vi "ListDQMH_HighLevel_VIs.vi"(2 "Filter":string[](array[string])=["Validate DQMH Module", "Rename DQMH Module"], 11 "error in":errorcluster) -> (4 "Events_Name":string[](array[string]), 6 "Events_Tag":string[](array[string]), 8 "Module_Name":string[](array[string]), 10 "Module_Tag":string[](array[string]), 15 "error IO":errorcluster)   [LabVIEW 2012]
panel:
  # "Connector Pane"
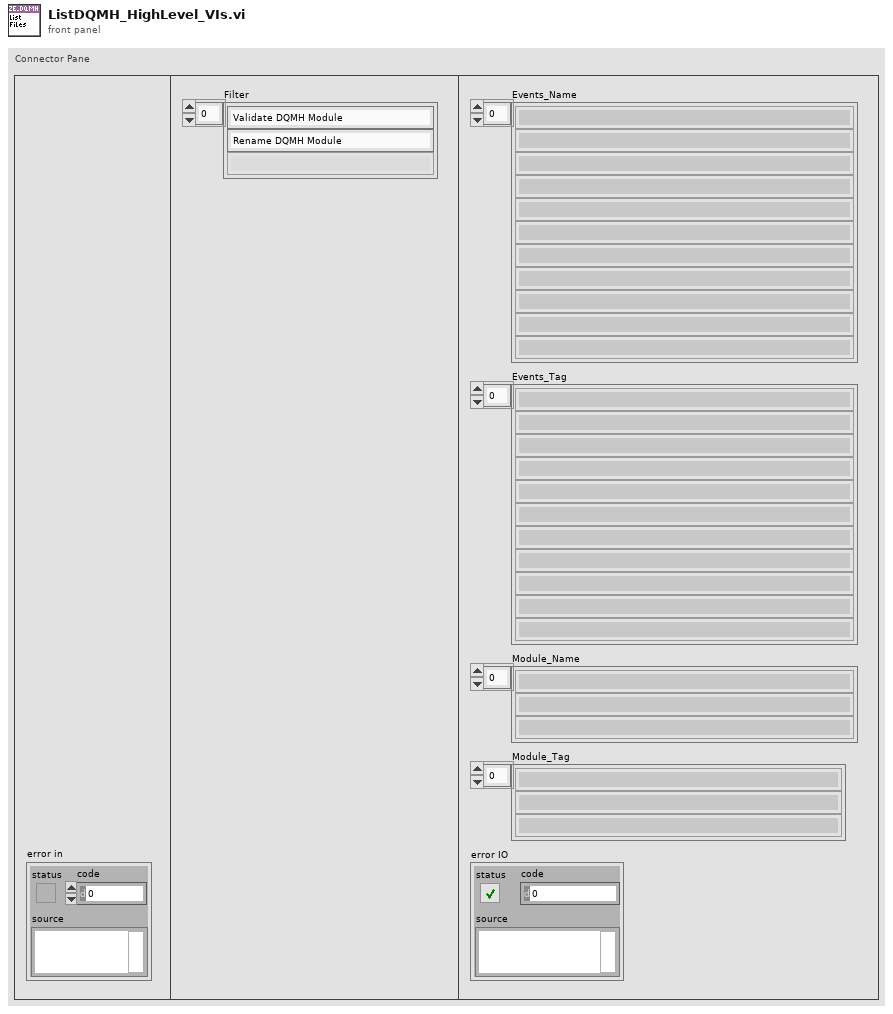
[diagram p1: front panel]
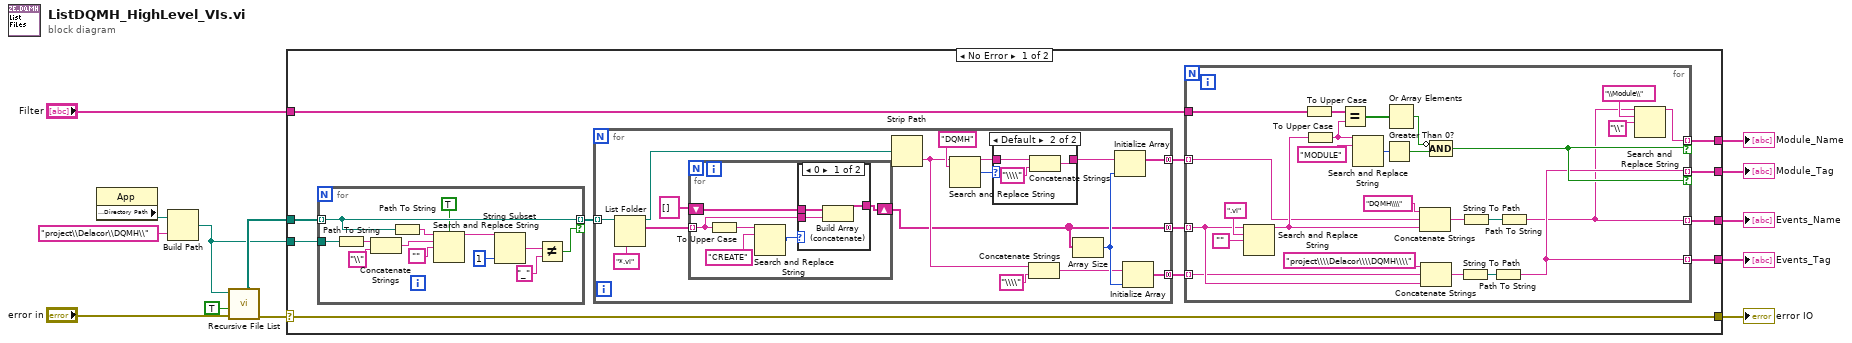
[diagram p0: block diagram]
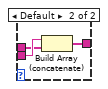
[diagram p2: hidden frame]
diagram:
  n1 = property class="App"() -> ("Application:Directory Path"=w11:path)  [unwired: 2 in, 2 out]
  n2 = Build Path(base path=w11, name or relative path="project\\Delacor\\DQMH\\") -> (appended path=w9:path)
  n3 = call <vilib>:"Recursive File List.vi"("error in (no error)"="error in", "Continue Recursing on Error? (F)"=TRUE, "Folder Path"=w9) -> ("error out"=w4:errorcluster, "All Folders"=w10:path[])  [unwired: 4 in, 3 out]
  n4 = case shown="No Error" w4 {
    selector: w4 -> [w18 w97]
    tunnel: w10 -> [w25 _]
    tunnel: w9 -> [w24 _]
    tunnel: [w21 _] -> w8
    tunnel: "Filter" -> [w20 _]
    tunnel: [w19 _] -> w1
    tunnel: [w18 w97] -> w5
    tunnel: [w17 _] -> w3
    tunnel: [w16 _] -> w2
    frame No Error {
      n5 = for {
        tunnel: w25 -> [w92] mode=indexing
        tunnel: [w92] -> w23 mode=indexing if=w93
        tunnel: w24 -> [w90]
        n6 = Path To String(path=w90) -> (string=w86:string)
        n7 = Concatenate Strings(w86, "\\" ("string")) -> (w85:string)
        n8 = Path To String(path=w92) -> (string=w91:string)
        n9 = Search and Replace String(case sensitive?=TRUE ("ignore case? (F)"), input string=w91, search string=w85, replace string="") -> (result string=w87:string)  [unwired: 4 in, 3 out]
        n10 = String Subset(string=w87, length (rest)=1 ("length (rest)")) -> (substring=w95:string)  [unwired: 1 in]
        n11 = Not Equal?(x=w95, y="_") -> (x != y?=w93:bool)
      }
      n12 = for {
        tunnel: w23 -> [w67] mode=indexing
        tunnel: [w52] -> w22 mode=concatenating
        tunnel: [w61] -> w15 mode=concatenating
        tunnel: [w56] -> w14 mode=concatenating
        n13 = List Folder(path=w67, pattern="*.vi") -> (path out=w59:path, filenames=w54:string[])  [unwired: 2 in, 2 out]
        n14 = for {
          tunnel: w54 -> [w71] mode=indexing
          shift-right: [w69] -> w52
          shift-left: string[] [] ("filenames") -> [w70]
          n15 = To Upper Case(1:w71) -> (0:w68:string)
          n16 = Search and Replace String(input string=w68, search string="CREATE") -> (number of replacements=w72:i32)  [unwired: 6 in, 3 out]
          n17 = case shown="0" w72 {
            tunnel: w71 -> [w76 w79]
            tunnel: w70 -> [w75 w78]
            tunnel: [w74 w77] -> w69
            frame 0 {
              n18 = Build Array (concatenate)(w75, w76) -> (w74:string[])
            }
            frame Default {
              n19 = Build Array (concatenate)(w79, w78) -> (w77:string[])
            }
          }
        }
        n20 = Strip Path(path=w59) -> (name=w55:string)  [unwired: 1 out]
        n21 = Search and Replace String(input string=w55, search string="DQMH") -> (result string=w63:string, number of replacements=w64:i32)  [unwired: 6 in, 2 out]
        n22 = case shown="Default" w64 {
          tunnel: w63 -> [w80 w83]
          tunnel: [w80 w81] -> w62
          frame 1.. {
          }
          frame Default {
            n23 = Concatenate Strings(w83, "\\\\" ("string")) -> (w81:string)
          }
        }
        n24 = Concatenate Strings(w55, "\\\\" ("string")) -> (w57:string)
        n25 = Array Size(array=w52) -> (size(s)=w60:i32)
        n26 = Initialize Array(w62, w60) -> (w61:string[])
        n27 = Initialize Array(w57, w60) -> (w56:string[])
      }
      n28 = for {
        tunnel: w22 -> [w36] mode=indexing
        tunnel: [w27] -> w21 mode=indexing
        tunnel: w20 -> [w48]
        tunnel: [w26] -> w19 mode=indexing if=w39
        tunnel: [w30] -> w17 mode=indexing if=w39
        tunnel: [w30] -> w16 mode=indexing
        tunnel: w15 -> [w37] mode=indexing
        tunnel: w14 -> [w35] mode=indexing
        n29 = Search and Replace String(input string=w36, search string=".vi", replace string="") -> (result string=w40:string)  [unwired: 5 in, 3 out]
        n30 = To Upper Case(1:w48) -> (0:w49:string[])
        n31 = To Upper Case(1:w40) -> (0:w46:string)
        n32 = Equal?(x=w49, y=w46) -> (x = y?=w47:bool[])
        n33 = Search and Replace String(input string=w46, search string="MODULE") -> (number of replacements=w44:i32)  [unwired: 6 in, 3 out]
        n34 = Greater Than 0?(x=w44) -> (x > 0?=w43:bool)
        n35 = Or Array Elements(Boolean array=w47) -> (logical OR=w42:bool)
        n36 = Concatenate Strings("DQMH\\\\" ("string"), w37, w40) -> (w34:string)
        n37 = Concatenate Strings("project\\\\Delacor\\\\DQMH\\\\" ("string"), w35, w36) -> (w33:string)
        n38 = Compound Arithmetic op=AND(invert w42, w43) -> (w39:bool)
        n39 = String To Path(string=w33) -> (path=w31:path)
        n40 = String To Path(string=w34) -> (path=w32:path)
        n41 = Path To String(path=w31) -> (string=w30:string)
        n42 = Path To String(path=w32) -> (string=w27:string)
        n43 = Search and Replace String(input string=w27, search string="\\Module\\", replace string="\\" ("replace string (\"\")")) -> (result string=w26:string)  [unwired: 5 in, 3 out]
      }
    }
    frame Error {
    }
  }
  "Events_Name" <- w8
  "Module_Name" <- w1
  "error IO" <- w5
  "Module_Tag" <- w3
  "Events_Tag" <- w2
